vi "CSM Not Found Error.vi"(8 "error in (no error)":errorcluster, 10 "Occured?":bool=TRUE, 11 "Queue Name":string) -> (0 "error out":errorcluster)   [LabVIEW 2017, in "Communicable State Machine.lvlib"]
uses:
  Communicable State Machine.lvlib
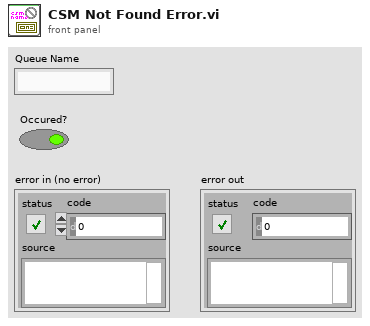
[diagram p1: front panel]
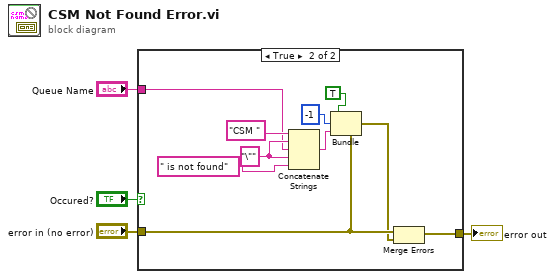
[diagram p0: block diagram]
diagram:
  n1 = case shown="True" "Occured?" {
    tunnel: "error in (no error)" -> [w5 w8]
    tunnel: [w5 w7] -> w2
    tunnel: "Queue Name" -> [_ w9]
    frame False {
    }
    frame True {
      w13 = "\"" ("string")
      n2 = Concatenate Strings("CSM " ("String to Prepend to source (\"\")"), w13, w9, w13, " is not found" ("string")) -> (w14:string)
      n3 = Bundle(cluster=w8, "status"=TRUE, "code"=-1, "source"=w14) -> (w6:errorcluster)
      n4 = Merge Errors(w8, w6) -> (w7:errorcluster)
    }
  }
  "error out" <- w2
